vi "VMI_save_delay_paths.vi"(4 "error in":errorcluster, 5 "Remote path 2":path, 6 "Delay_full_dir":string[](array[string]), 7 "Main Directory":path) -> (0 "error out":errorcluster, 1 "appended path":path, 2 "Delay_paths":path[](array[path]), 3 "New Date Name":string)   [LabVIEW 2019]
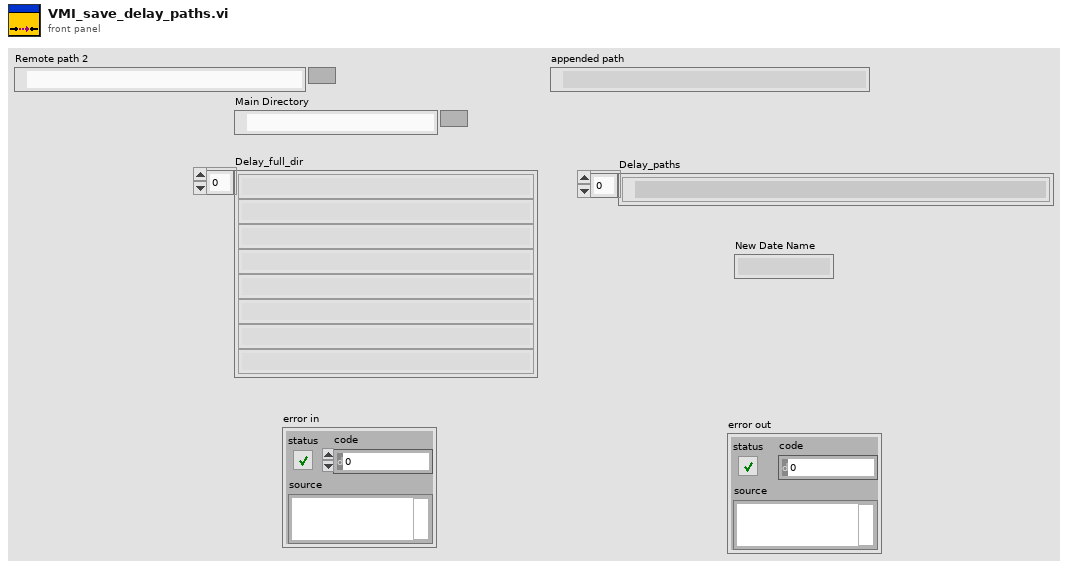
[diagram p1: front panel]
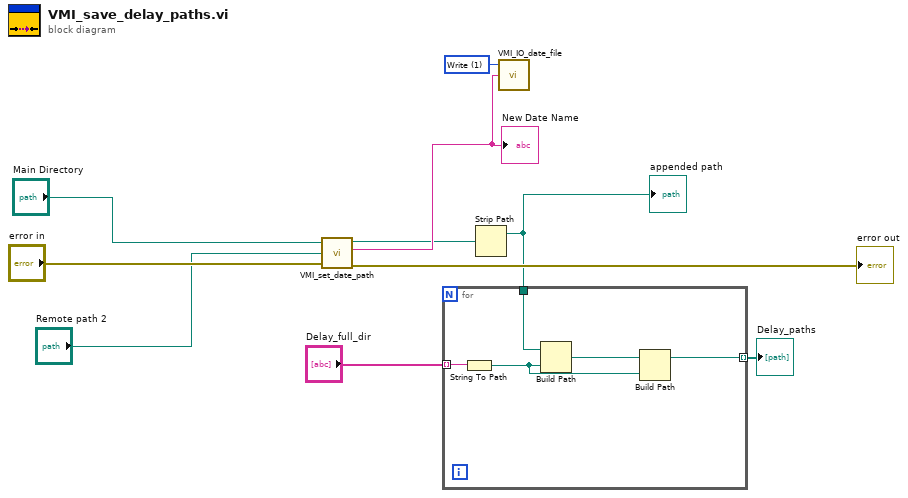
[diagram p0: block diagram]
diagram:
  w4 = u16 1 items=["Read", "Write"] ("File Task")
  n1 = call "VMI_set_date_path.vi"("Value"="Main Directory", "Remote path 2"="Remote path 2", "error in (no error)"="error in") -> ("appended path"=w2:path, "New Date Name"=w3:string, "error out"=→"error out":errorcluster)  [unwired: 1 out]
  "New Date Name" <- w3
  n2 = Strip Path(path=w2) -> (stripped path=w1:path)  [unwired: 1 out]
  "appended path" <- w1
  n3 = for {
    tunnel: "Delay_full_dir" -> [w15] mode=indexing
    tunnel: w1 -> [w14]
    tunnel: [w11] -> w7 mode=indexing
    n4 = String To Path(string=w15) -> (path=w13:path)
    n5 = Build Path(base path=w14, name or relative path=w13) -> (appended path=w12:path)
    n6 = Build Path(base path=w12, name or relative path=w13) -> (appended path=w11:path)
  }
  "Delay_paths" <- w7
  n7 = call "VMI_IO_date_file.vi"("File date in"=w3, "File Task"=w4) -> ()  [unwired: 2 in, 2 out]
